vi "Start.vi"(8 "error in":errorcluster, 11 "PCAN Basic in":refnum<class "PCAN Basic Base Configure Strategy.lvclass">) -> (0 "error out":errorcluster, 3 "PCAN Basic out":refnum<class "PCAN Basic Base Configure Strategy.lvclass">)   [LabVIEW 2025, in "PCAN Basic Base Configure Strategy.lvclass"]
uses:
  PCAN Basic Base Configure Strategy.lvclass
  PCAN Basic Base Configure Strategy.lvclass/PCAN Basic Base Configure Strategy.ctl
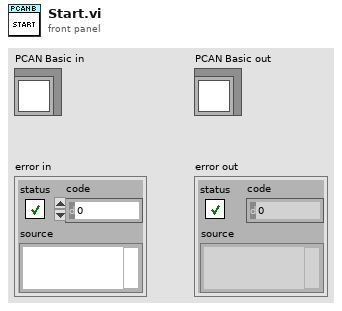
[diagram p1: front panel]
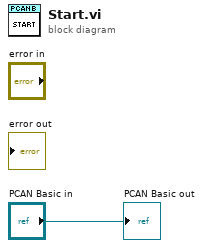
[diagram p0: block diagram]
diagram:
  "PCAN Basic out" <- "PCAN Basic in"
